vi "Set RefrigCapacity.vi"(7 "Capacity set point (0-9)":i32 min=0 max=9 step=1, 8 "error in (no error)":errorcluster, 10 "Address (0)":i32, 11 "VISA resource name":refnum<visa-resource-name>) -> (0 "error out":errorcluster, 3 "VISA resource name out":refnum<visa-resource-name>)   [LabVIEW 2021, in "Environment Chamber.lvlib" / "Climatic Chamber.lvlib"]
doc: "<b>Refrigerator-related settings</b>\n\nChanges the refrigeration capacity set point in constant mode No. 1\n\n<b>P200:</B>\nEnter 0 to 9 for the set point.\nSet point 0: Manual OFF (Stop)\nSet point 1: Manual ON\nSet point 2 to 9: Auto\n\n<b>SCP-220, P300:</B>\nEnter 0 to 9 for the set point.\nSet point 0: Manual OFF (Stop)\nSet point 1 to 2: Manual 20% (Output: Small)\nSet point 3 to 5: Manual 50% (Output: Medium)\nSet point 6 to 8: Manual 100% (Max. Output)\nSet point 9: Auto"
uses:
  Climatic Chamber.lvlib
panel:
  out "NACK":bool
  out "Error":bool
  out "ACK":bool
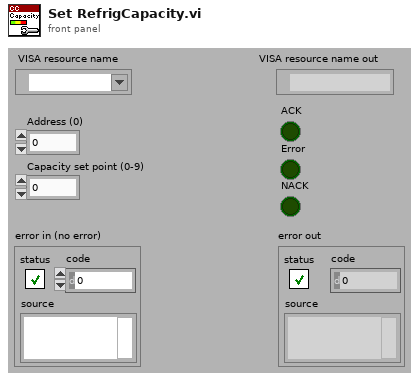
[diagram p1: front panel]
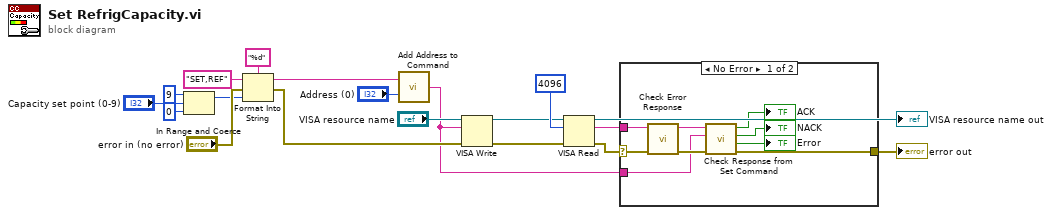
[diagram p0: block diagram]
diagram:
  n1 = In Range and Coerce(upper limit=9, x="Capacity set point (0-9)", lower limit=0) -> (coerced(x)=w3:i32)  [unwired: 1 out]
  n2 = Format Into String(format string="%d", initial string="SET,REF", error in="error in (no error)", w3) -> (resulting string=w6:string, error out=w5:errorcluster)
  n3 = call "Add Address to Command.vi"("Address (0)"="Address (0)", "Command"=w6) -> ("Command OUT"=w4:string)
  n4 = VISA Write(VISA resource name="VISA resource name", write buffer=w4, error in (no error)=w5) -> (VISA resource name out=w16:refnum<visa-resource-name>, error out=w15:errorcluster)  [unwired: 1 out]
  n5 = VISA Read(VISA resource name=w16, byte count=u32 4096, error in (no error)=w15) -> (VISA resource name out=→"VISA resource name out":refnum<visa-resource-name>, read buffer=w11:string, error out=w12:errorcluster)  [unwired: 1 out]
  n6 = case shown="No Error" w12 {
    selector: w12 -> [w27 w29]
    tunnel: w11 -> [w28 _]
    tunnel: [w23 w29] -> w10
    tunnel: w4 -> [w24 _]
    frame No Error {
      n7 = call "Check Error Response.vi"("error in (no error)"=w27, "read String"=w28) -> ("error out"=w26:errorcluster, "String out"=w25:string)  [unwired: 7 in, 1 out]
      n8 = call "Check Response from Set Command.vi"("error in (no error)"=w26, "Command"=w24, "Response"=w25) -> ("error out"=w23:errorcluster, "Error"=→"Error":bool, "NACK"=→"NACK":bool, "ACK"=→"ACK":bool)  [unwired: 5 in]
    }
    frame Error {
    }
  }
  "error out" <- w10
